vi "Set Value By Name.vi"(8 "error in (no error)":errorcluster, 9 "Value":variant, 10 "Name":string, 11 "LUT in":refnum<class "LUT.lvclass">) -> (0 "error out":errorcluster, 2 "found?":bool, 3 "LUT out":refnum<class "LUT.lvclass">)   [LabVIEW 2017, in "LUT.lvlib" / "LUT.lvclass"]
doc: "Changes or creates an attribute name and value."
uses:
  LUT.lvclass
  LUT.lvclass/LUT.ctl
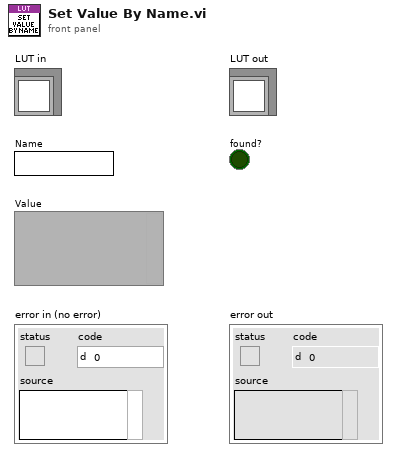
[diagram p1: front panel]
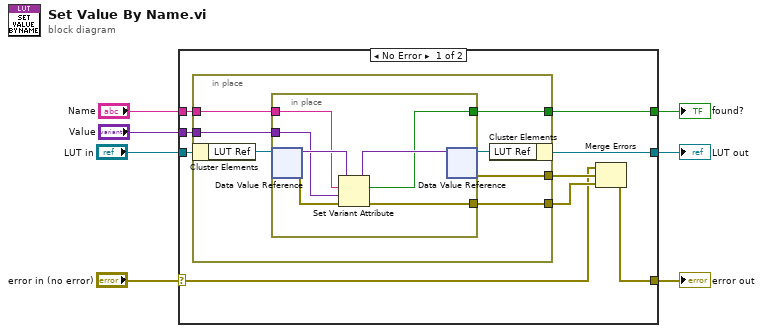
[diagram p0: block diagram]
diagram:
  n1 = case shown="No Error" "error in (no error)" {
    selector: "error in (no error)" -> [w10 w32]
    tunnel: [w9 w32] -> w6
    tunnel: [w15 w31] -> w4
    tunnel: "LUT in" -> [w16 w31]
    tunnel: "Name" -> [w14 _]
    tunnel: [w13 _] -> w2
    tunnel: "Value" -> [w8 _]
    frame No Error {
      n2 = in-place {
        in-place-border: w14 -> [w21]
        in-place-border: [w20] -> w13
        in-place-border: [w19] -> w11
        in-place-border: [w18] -> w12
        in-place-border: w8 -> [w17]
        n3 = in-place-cluster #1(w16) -> ("LUT Ref"=w23:refnum<data-value>)
        n4 = in-place {
          in-place-border: w21 -> [w29]
          in-place-border: [w24] -> w20
          in-place-border: [w27] -> w19
          in-place-border: w17 -> [w26]
          n5 = in-place-dvr #2(w23) -> (w30:variant, w28:errorcluster)
          n6 = Set Variant Attribute(Variant=w30, name=w29, value=w26, error in=w28) -> (Variant out=w25:variant, replaced=w24:bool, error out=w27:errorcluster)
          n7 = in-place-dvr #2(w25) -> (w22:refnum<data-value>, w18:errorcluster)
        }
        n8 = in-place-cluster #1("LUT Ref"=w22) -> (w15:refnum<class "LUT.lvclass">)
      }
      n9 = Merge Errors(w10, w12, w11) -> (w9:errorcluster)
    }
    frame Error {
    }
  }
  "error out" <- w6
  "LUT out" <- w4
  "found?" <- w2
